vi "uActor_Exec.vi"(6 "Original uMsg":refnum<class "uMsg.lvclass">, 8 "error in (no error)":errorcluster, 9 "Data":refnum<class "uData.lvclass">, 10 "Command":string, 11 "uBroker in":refnum<class "uBroker.lvclass">) -> (0 "error out":errorcluster, 1 "reply":refnum<class "uData.lvclass">, 3 "uBroker out":refnum<class "uBroker.lvclass">)   [LabVIEW 2023, in "uLib.lvlib" / "uBroker.lvclass"]
uses:
  uBroker.lvclass
  uData/uData/uData.lvclass
  uMsg/uMsg/uMsg.lvclass
  uData/uData/uData.lvclass/uData.ctl
  uBroker.lvclass/uBroker.ctl
  uMsg/uMsg/uMsg.lvclass/uMsg.ctl
  uData/uData/Condition Tag Name.vi
  uData/uData/Combine Tags.vi
  uTransport/uTransport/uTransport_SendMsg.vi
  uData/uData/Blank Key Reserved String.vi
  uMsg/uMsg/uMsg Update Timestamp.vi
  uTransport/uTransport/uTransport.lvclass
  uActor/uActor/uActor.lvclass
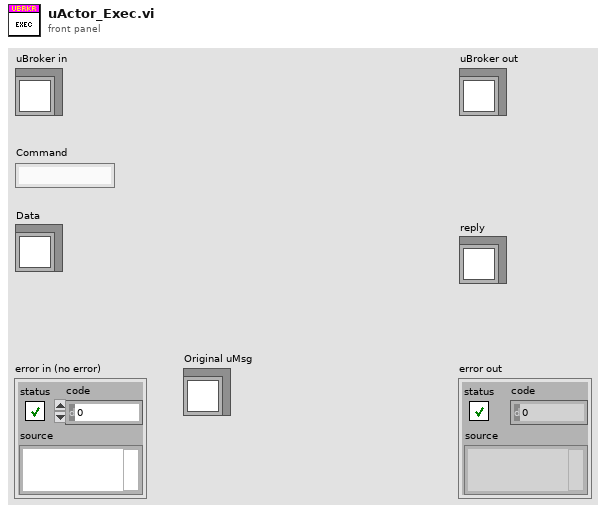
[diagram p1: front panel]
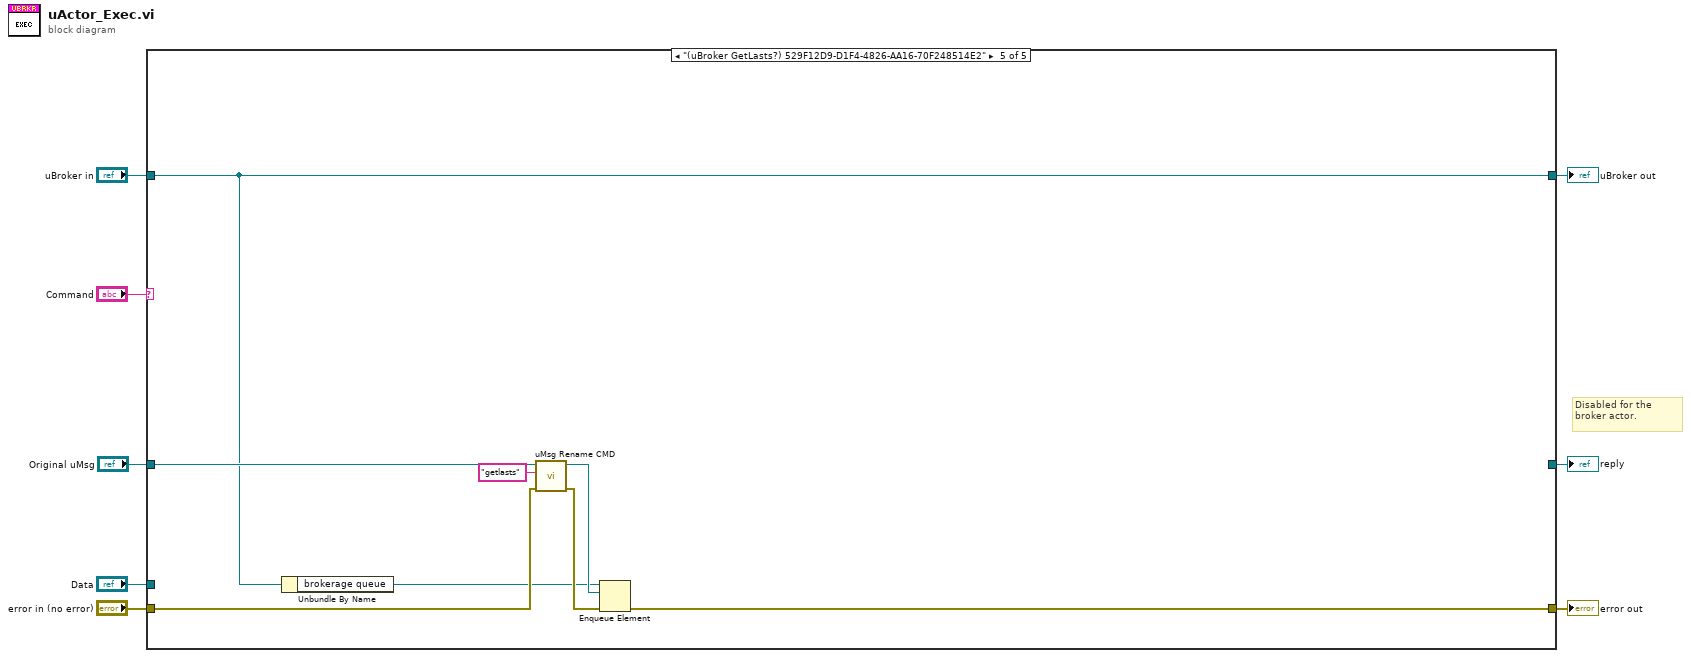
[diagram p0: block diagram]
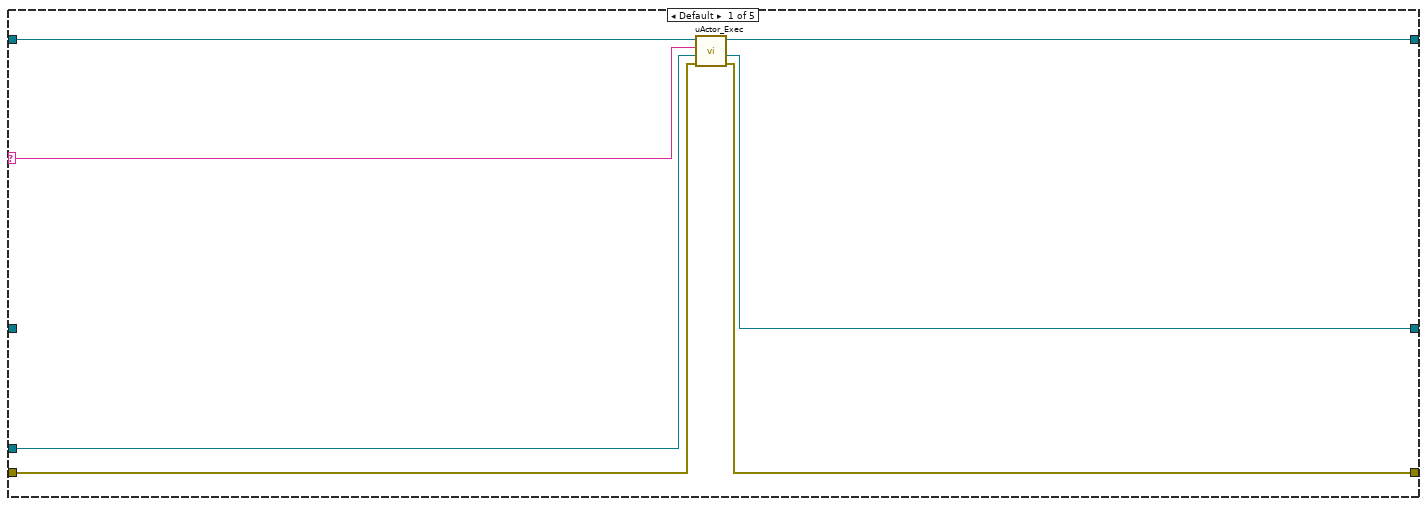
[diagram p2: hidden frame]
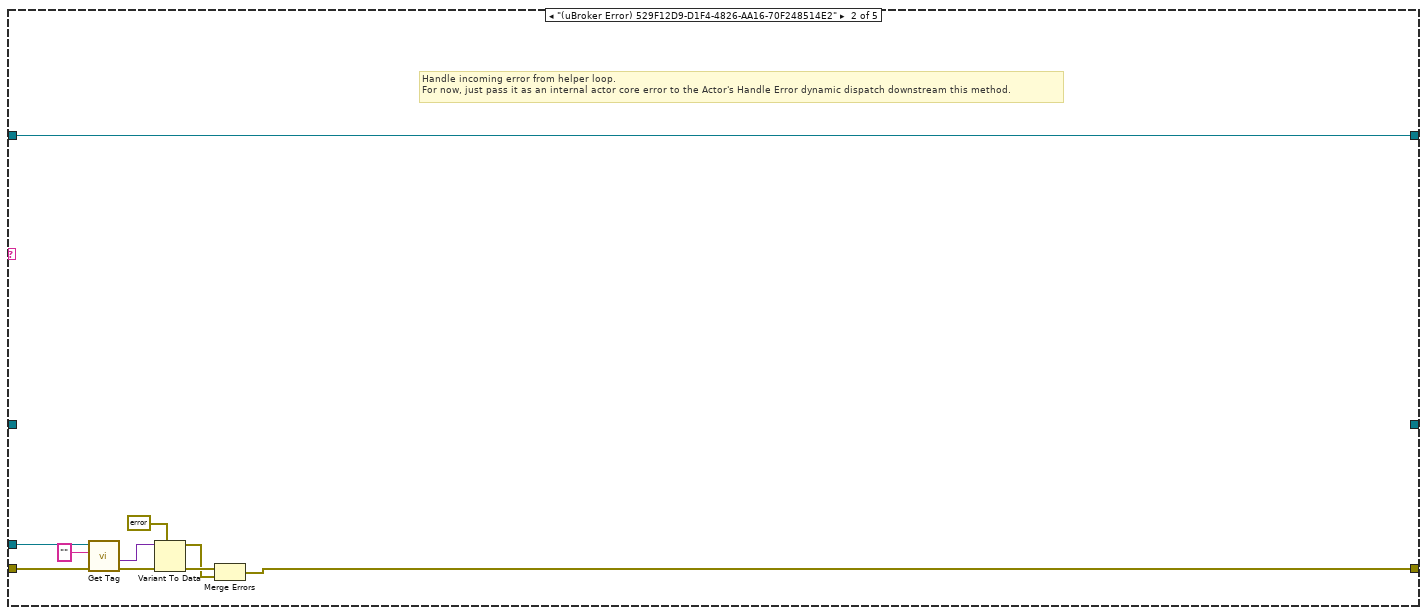
[diagram p3: hidden frame]
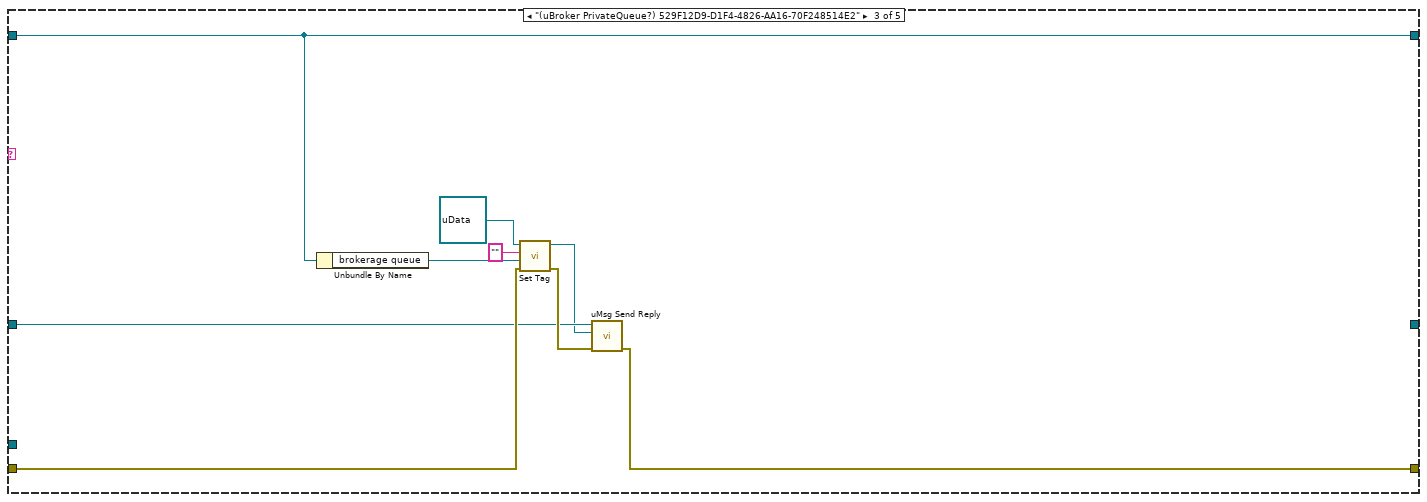
[diagram p4: hidden frame]
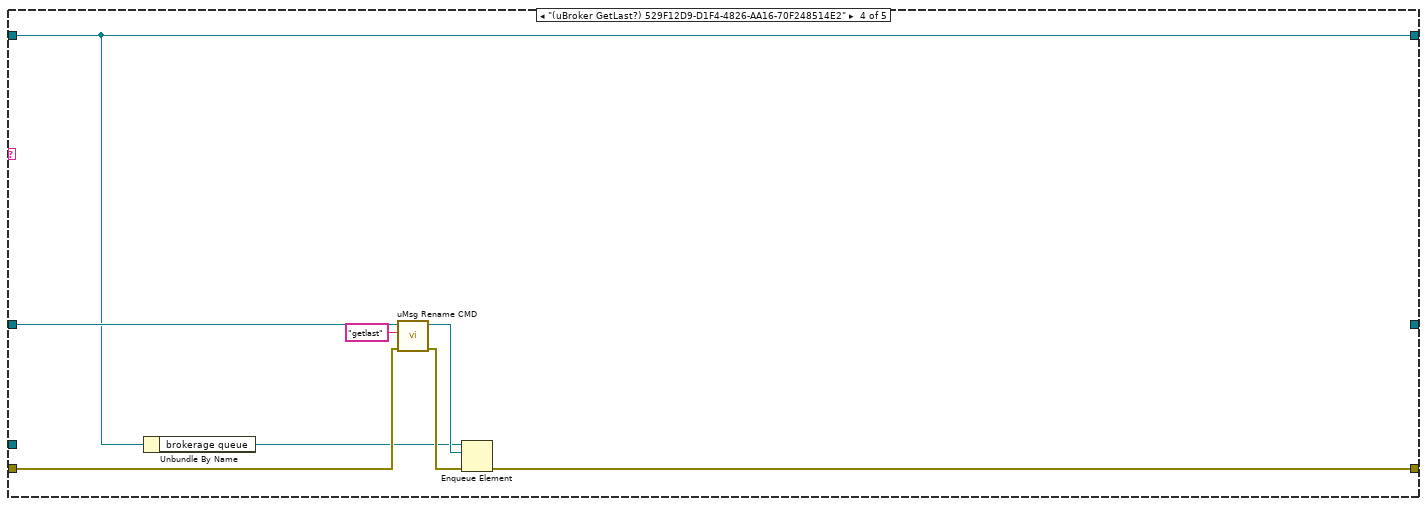
[diagram p5: hidden frame]
diagram:
  # "Disabled for the broker actor."
  n1 = case shown="\"(uBroker GetLasts?) 529F12D9-D1F4-4826-AA16-70F248514E2\"" "Command" {
    selector: "Command" -> [w10 _ _ _ _]
    tunnel: [w15 w25 w33 w39 w47] -> w8
    tunnel: "Data" -> [w14 w24 _ _ _]
    tunnel: "uBroker in" -> [w13 w25 w33 w39 w47]
    tunnel: "error in (no error)" -> [w12 w20 w31 w41 w49]
    tunnel: [w11 w18 w26 w37 w45] -> w3
    tunnel: [w9 _ _ _ _] -> w2
    tunnel: "Original uMsg" -> [_ _ w28 w42 w50]
    frame Default {
      n2 = call-parent "uActor_Exec.vi"("error in (no error)"=w12, "Data"=w14, "Command"=w10, "uActor in"=w13) -> ("error out"=w11:errorcluster, "reply"=w9:refnum<class "uData.lvclass">, "uActor out"=w15:refnum<class "uBroker.lvclass">)  [unwired: 5 in]
    }
    frame "(uBroker Error) 529F12D9-D1F4-4826-AA16-70F248514E2" {
      # "Handle incoming error from helper loop.\nFor now, just pass it as an internal actor core error to the Actor's Handle Error dynamic dispatch downstream this method."
      n3 = call "Get Tag.vi"("error in (no error)"=w20, "tag (case insensitive)"="", "uData in"=w24) -> ("error out"=w22:errorcluster, "value"=w21:variant)  [unwired: 5 in, 2 out]
      n4 = Variant To Data(error in=w22, type=errorcluster {"status"=FALSE, "code"=0, "source"=""} ("error out"), Variant=w21) -> (data=w17:errorcluster, error out=w19:errorcluster)
      n5 = Merge Errors(w19, w17) -> (w18:errorcluster)
    }
    frame "(uBroker PrivateQueue?) 529F12D9-D1F4-4826-AA16-70F248514E2" {
      n6 = Unbundle By Name(w33) -> ("brokerage queue"=w32:refnum<queue>)
      n7 = call "Set Tag.vi"("error in (no error)"=w31, "Variant"=w32, "tag (case insensitive)"="", "uData in"=refnum<class "uData.lvclass"> refnum) -> ("error out"=w34:errorcluster, "uData out"=w27:refnum<class "uData.lvclass">)  [unwired: 5 in, 1 out]
      n8 = call "uMsg Send Reply.vi"("error in (no error)"=w34, "Reply Data"=w27, "Original Msg"=w28) -> ("error out"=w26:errorcluster)  [unwired: 8 in]
    }
    frame "(uBroker GetLast?) 529F12D9-D1F4-4826-AA16-70F248514E2" {
      n9 = Unbundle By Name(w39) -> ("brokerage queue"=w35:refnum<queue>)
      n10 = call "uMsg Rename CMD.vi"("error in (no error)"=w41, "New CMD"="getlast", "uMsg in"=w42) -> ("error out"=w40:errorcluster, "uMsg out"=w36:refnum<class "uMsg.lvclass">)  [unwired: 7 in]
      n11 = Enqueue Element(queue=w35, element=w36, error in (no error)=w40) -> (error out=w37:errorcluster)  [unwired: 1 in, 2 out]
    }
    frame "(uBroker GetLasts?) 529F12D9-D1F4-4826-AA16-70F248514E2" {
      n12 = Unbundle By Name(w47) -> ("brokerage queue"=w43:refnum<queue>)
      n13 = call "uMsg Rename CMD.vi"("error in (no error)"=w49, "New CMD"="getlasts", "uMsg in"=w50) -> ("error out"=w48:errorcluster, "uMsg out"=w44:refnum<class "uMsg.lvclass">)  [unwired: 7 in]
      n14 = Enqueue Element(queue=w43, element=w44, error in (no error)=w48) -> (error out=w45:errorcluster)  [unwired: 1 in, 2 out]
    }
  }
  "error out" <- w3
  "uBroker out" <- w8
  "reply" <- w2
